vi "Sync Project Config.vi"(8 "Error In":errorcluster, 11 "Sync Source Config":T1) -> (0 "Error Out":errorcluster, 3 "Sync Source Config":T1)   [LabVIEW 2011, in "LVH-Build-Tools.lvlib"]
doc: "Load configuration values from ini and allow user to change and save values."
uses:
  <vilib>/LabVIEW Hacker/Build Tools/LVH-Build-Tools.lvlib
  Type Defs/Sync Source Configuration.ctl
  Type Defs/Installed Project.ctl
  Local Toolbox/_Installed LabVIEW Version.ctl
panel:
  in  "Project Backup Dir":path
  in  "Save Button":bool
  in  "Cancel Button":bool
  in  "Project Source Root Directory":path
  # "LVH Build Tools Configuration\n\nPlease select the project source root directory and a directory to \nstore backup archives."
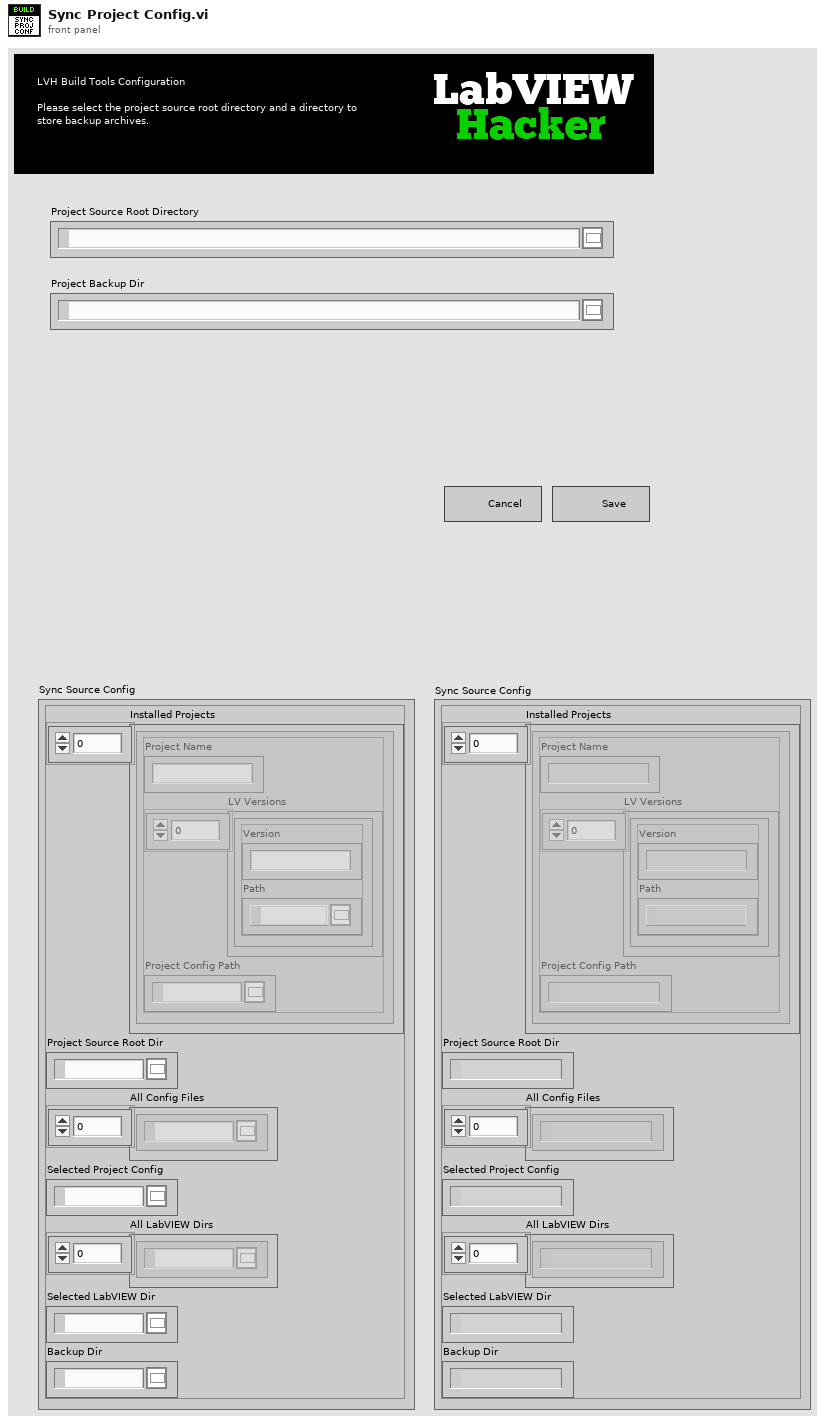
[diagram p1: front panel]
types:
  T1 = typedef "LVH-Build-Tools.lvlib/Sync Source Configuration.ctl" = cluster{"Installed Projects":T2[], "Project Source Root Dir":path, "All Config Files":path[], "Selected Project Config":path, "All LabVIEW Dirs":path[], "Selected LabVIEW Dir":path, "Backup Dir":path}
  T2 = typedef "LVH-Build-Tools.lvlib/Installed Project.ctl" = cluster{"Project Name":string, "LV Versions":T3[], "Project Config Path":path}
  T3 = typedef "LVH-Build-Tools.lvlib/_Installed LabVIEW Version.ctl" = cluster{"Version":string, "Path":path}
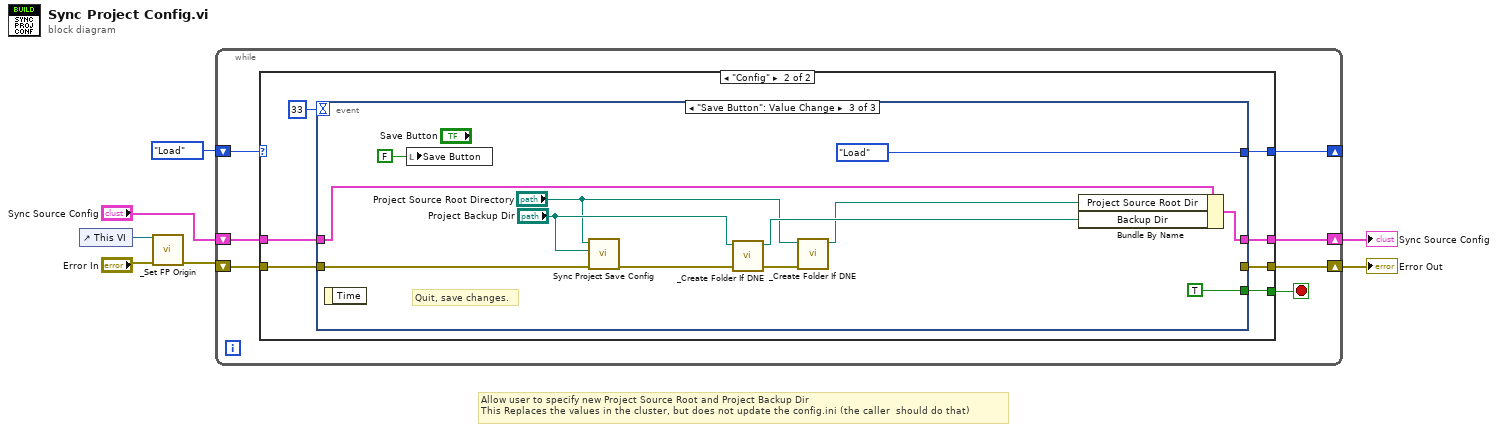
[diagram p0: block diagram]
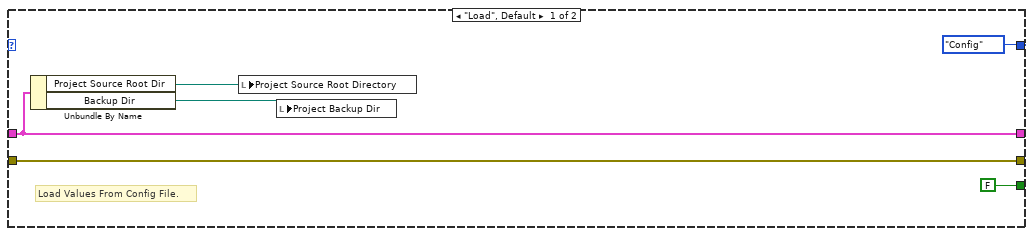
[diagram p2: hidden frame]
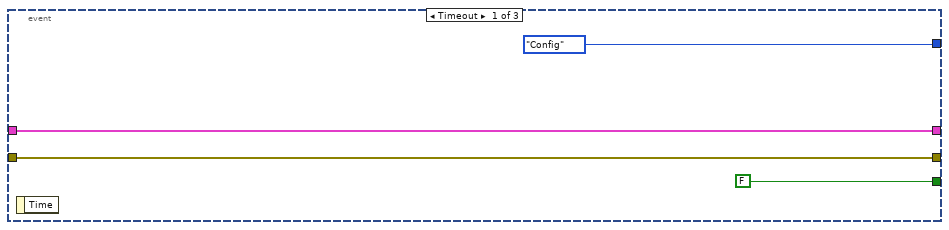
[diagram p3: hidden frame]
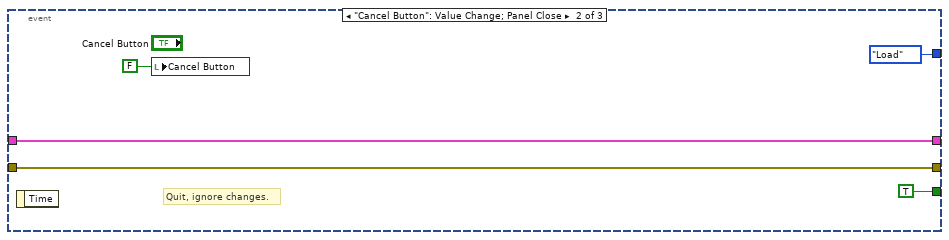
[diagram p4: hidden frame]
diagram:
  # "Allow user to specify new Project Source Root and Project Backup Dir\nThis Replaces the values in the cluster, but does not update the config.ini (the caller  should do that)"
  n1 = control-ref of="This VI"() -> (w3:refnum<vi>)
  n2 = call "_Set FP Origin.vi"("Error In"="Error In", "VI Ref"=w3) -> ("Error Out"=w2:errorcluster)  [unwired: 9 in]
  n3 = while {
    shift-right: [w11] -> w1
    shift-left: w2 -> [w13]
    shift-right: [w12] -> _
    shift-left: enum16{"Load", "Config"}."Load" ("Sync Project Config State") -> [w14]
    shift-right: [w8] -> w5
    shift-left: "Sync Source Config" -> [w9]
    stop <- w10 stop-if-true
    n4 = case shown="\"Config\"" w14 {
      tunnel: w13 -> [w16 w24]
      tunnel: [enum16{"Load", "Config"}."Config" ("Sync Project Config State") w26] -> w12
      tunnel: [w16 w25] -> w11
      tunnel: [FALSE w23] -> w10
      tunnel: w9 -> [w15 w22]
      tunnel: [w15 w21] -> w8
      frame "Load", Default {
        # "Load Values From Config File."
        n5 = Unbundle By Name(w15) -> ("Project Source Root Dir"=w17:path, "Backup Dir"=w18:path)
        n6 = local write "Project Source Root Directory"(w17) -> ()
        n7 = local write "Project Backup Dir"(w18) -> ()
      }
      frame "Config" {
        n8 = event shown="[2] \"Save Button\": Value Change" {
          selector: _ -> [_ _ _]
          dyn-events: _ -> [_ _ _]
          timeout: 33 -> [_ _ _]
          tunnel: [enum16{"Load", "Config"}."Config" ("Sync Project Config State") enum16{"Load", "Config"}."Load" ("Sync Project Config State") enum16{"Load", "Config"}."Load" ("Sync Project Config State")] -> w26
          tunnel: [w30 w33 _] -> w25
          tunnel: w24 -> [w30 w33 w45]
          tunnel: [FALSE TRUE TRUE] -> w23
          tunnel: w22 -> [w28 w32 w42]
          tunnel: [w28 w32 w40] -> w21
          event Timeout {
            n9 = event-data() -> ()  [unwired: 1 in, 1 out]
          }
          event "Cancel Button": Value Change; Panel Close {
            # "Quit, ignore changes."
            n10 = event-data() -> ()  [unwired: 1 in, 1 out]
            n11 = local write "Cancel Button"(FALSE ("Cancel Button")) -> ()
          }
          event "Save Button": Value Change {
            # "Quit, save changes."
            n12 = event-data() -> ()  [unwired: 1 in, 1 out]
            n13 = local write "Save Button"(FALSE ("Save Button")) -> ()
            n14 = call "Sync Project Save Config.vi"("Error In"=w45, "Project Backup Archive Directory"="Project Backup Dir", "Project Source Root Directory"="Project Source Root Directory") -> ("Error Out"=w44:errorcluster)  [unwired: 8 in]
            n15 = call "_Create Folder If DNE.vi"("Error In"=w44, "Folder Path"="Project Backup Dir") -> ("Error Out"=w39:errorcluster, "Dup Path"=w41:path)  [unwired: 8 in]
            n16 = call "_Create Folder If DNE.vi"("Error In"=w39, "Folder Path"="Project Source Root Directory") -> ("Dup Path"=w37:path)  [unwired: 8 in, 1 out]
            n17 = Bundle By Name(cluster=w42, "Project Source Root Dir"=w37, "Backup Dir"=w41) -> (w40:T1)
          }
        }
      }
    }
  }
  "Error Out" <- w1
  "Sync Source Config" <- w5
